vi "DB_Execute_Query.vi"() -> ()   [LabVIEW 2020]
uses:
  <vilib>/addons/database/Connection.llb/DB Tools Open Connec (String).vi
  <vilib>/addons/database/Connection.llb/Conn Execute.vi
  <vilib>/addons/database/Recordset.llb/Rec Fetch Recordset Data (R).vi
  <vilib>/addons/database/Recordset.llb/Rec Destroy - Connection.vi
  <vilib>/addons/database/NI_Database_API.lvlib
panel:
  out "recordset data":variant[][](array[variant])
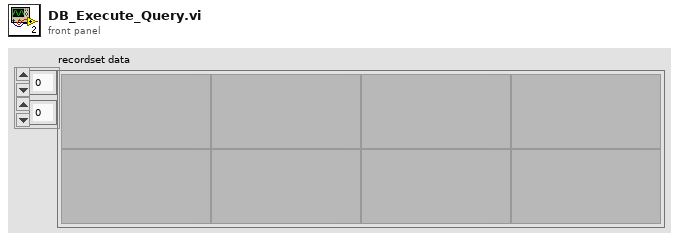
[diagram p1: front panel]
types:
  T1 = typedef "NI_Database_API.lvlib/Conn ObjectReference.ctl" = refnum<k1>
  T2 = typedef "NI_Database_API.lvlib/Rec ObjectReference.ctl" = refnum<k1>
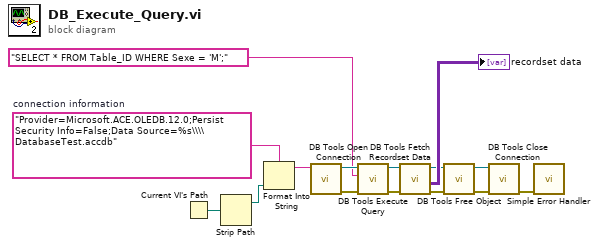
[diagram p0: block diagram]
diagram:
  w8 = "Provider=Microsoft.ACE.OLEDB.12.0;Persist Security Info=False;Data Source=%s\\\\DatabaseTest.accdb"  # connection information
  n1 = Current VI's Path() -> (path=w12:path)
  n2 = Strip Path(path=w12) -> (stripped path=w9:path)  [unwired: 1 out]
  n3 = Format Into String(format string=w8, w9) -> (resulting string=w10:string)  [unwired: 2 in, 1 out]
  n4 = call-poly <vilib>:"DB Tools Open Connection.vi"("connection information"=w10) -> ("error out"=w14:errorcluster, "connection reference"=w15:T1)  [unwired: 7 in]
  n5 = call-poly <vilib>:"DB Tools Execute Query.vi"("error in (no error)"=w14, "SQL query"="SELECT * FROM Table_ID WHERE Sexe = 'M';", "connection reference"=w15) -> ("error out"=w4:errorcluster, "recordset reference"=w3:T2)  [unwired: 5 in]
  n6 = call-poly <vilib>:"DB Tools Fetch Recordset Data.vi"("error in (no error)"=w4, "recordset reference"=w3) -> ("error out"=w1:errorcluster, "recordset data"=→"recordset data":variant[][], "recordset reference out"=w2:T2)  [unwired: 3 in]
  n7 = call-poly <vilib>:"DB Tools Free Object.vi"("error in (no error)"=w1, "recordset reference"=w2) -> ("error out"=w7:errorcluster, "connection reference"=w13:T1)  [unwired: 8 in]
  n8 = call <vilib>:"DB Tools Close Connection.vi"("error in (no error)"=w7, "connection reference"=w13) -> ("error out"=w11:errorcluster)  [unwired: 5 in]
  n9 = call <vilib>:"Simple Error Handler.vi"("error in (no error)"=w11) -> ()  [unwired: 4 in, 5 out]
